vi "Reorder.vi"(11 "POTTypedCircularBuffer in":refnum<class "ErrorLogBuffer.lvclass">) -> (3 "POTTypedCircularBuffer out":refnum<class "ErrorLogBuffer.lvclass">)   [LabVIEW 2024, in "ErrorLogBuffer.lvclass"]
doc: "rotate array so that the tail is at the 0th index"
uses:
  ErrorLogBuffer.lvclass
  ErrorLogBuffer.lvclass/ErrorLogBuffer.ctl
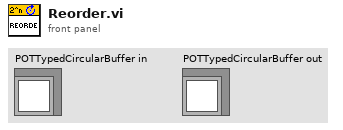
[diagram p1: front panel]
types:
  T1 = typedef "ErrorLogBuffer.lvclass/Type.ctl" = refnum<class "LogRecord.lvclass">
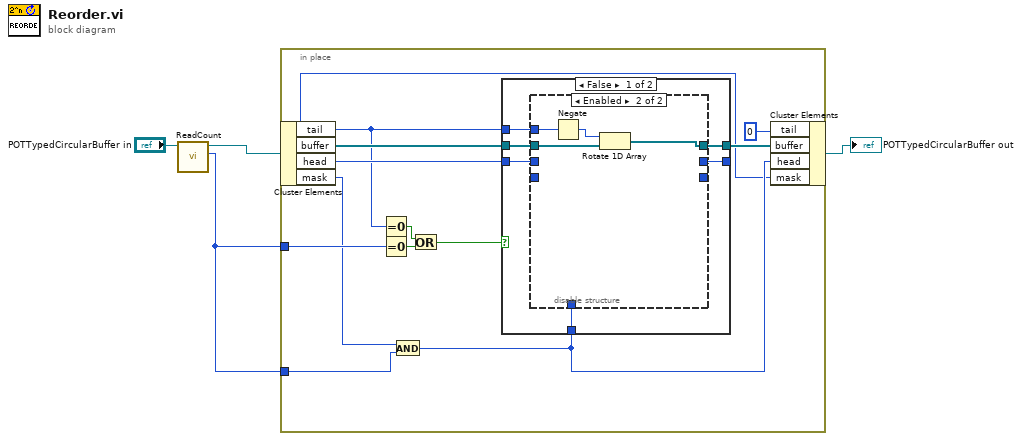
[diagram p0: block diagram]
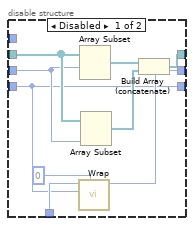
[diagram p2: hidden frame]
diagram:
  n1 = call "ReadCount.vi"("POTTypedCircularBuffer in"="POTTypedCircularBuffer in") -> ("count"=w1:i32, "POTTypedCircularBuffer out"=w2:refnum<class "ErrorLogBuffer.lvclass">)  [unwired: 9 in]
  n2 = in-place {
    in-place-border: w1 -> [w7]
    in-place-border: w1 -> [w12]
    n3 = in-place-cluster #1(w2) -> ("tail"=w10:i32, "buffer"=w16:T1[], "head"=w14:i32, "mask"=w5:i32)
    n4 = Equal To 0?(x=w10) -> (x = 0?=w9:bool)
    n5 = Equal To 0?(x=w12) -> (x = 0?=w11:bool)
    n6 = And(x=w5, y=w7) -> (x .and. y?=w6:i32)
    n7 = Or(x=w9, y=w11) -> (x .or. y?=w8:bool)
    n8 = case shown="False" w8 {
      tunnel: w16 -> [w21 w37]
      tunnel: [w22 w37] -> w15
      tunnel: w14 -> [w20 w36]
      tunnel: w10 -> [w17 _]
      tunnel: w6 -> [w19 _]
      tunnel: [w18 w36] -> _
      frame False {
        n9 = disable-structure shown="Enabled" {
          disable-tunnel: [w31 w33] -> w22
          disable-tunnel: w21 -> [w30 w35]
          disable-tunnel: w20 -> [w29 _]
          disable-tunnel: _ -> [w23 _]
          disable-tunnel: w19 -> [w25 _]
          disable-tunnel: [w24 _] -> w18
          disable-tunnel: w17 -> [_ w32]
          disable-tunnel: [w23 _] -> _
          frame Disabled {
            n10 = call "Wrap.vi"("increment amount (1)"=0 ("index"), "mask"=w23, "index"=w25) -> ("wrapped"=w24:i32)  [unwired: 8 in]
            n11 = Array Subset(array=w30, index=w29) -> (w28:T1[])  [unwired: 1 in]
            n12 = Array Subset(array=w30, length=w29) -> (w27:T1[])  [unwired: 1 in]
            n13 = Build Array (concatenate)(w28, w27) -> (w31:T1[])
          }
          frame Enabled {
            n14 = Negate(x=w32) -> (-x=w34:i32)
            n15 = Rotate 1D Array(1:w35, 2:w34) -> (0:w33:T1[])
          }
        }
      }
      frame True {
      }
    }
    n16 = in-place-cluster #1("tail"=0 ("head"), "buffer"=w15, "head"=w6, "mask"=w5) -> (→"POTTypedCircularBuffer out":refnum<class "ErrorLogBuffer.lvclass">)
  }
